vi "6704_set_static_voltages.vi"(6 "error in":errorcluster, 8 "6704 Static Voltage Settings":T1={"Device Name"="6704_Static", "Values"=[5.0, 0.0, 0.0, 0.0, 0.0, 0.0, 0.0, 0.0, 0.0, 0.0, 0.0, 0.0, 0.0, 0.0, 0.0, 0.0], "Nickname"=["", "", "", "", "", "", "", "", "", "", "", "", "", "", "", ""], "Conversion"=[enum."Volts", enum."Volts", enum."Volts", enum."Volts", enum."Volts", enum."Volts", enum."Volts", enum."Volts", enum."Volts", enum."Volts", enum."Volts", enum."Volts", enum."Volts", enum."Volts", enum."Volts", enum."Volts"]}) -> (0 "error out":errorcluster, 2 "Voltages Out":dbl[](array[numeric]))   [LabVIEW 2015]
uses:
  Controls/6704/6704_static_voltages_control.ctl
  Controls/6704/static_voltage_conversions.ctl
  Controls/6704/6704_state_machine_enum.ctl
  <vilib>/DAQmx/write.llb/DAQmx Write (Analog 1D DBL NChan 1Samp).vi
  <vilib>/DAQmx/create/channels.llb/DAQmx Create Channel (AO-Voltage-Basic).vi
  <vilib>/DAQmx/miscellaneous.llb/DAQmx Fill In Error Info.vi
  <resource>/objmgr/daqmx.rc
panel:
  out "AO.Voltage.Rngs":dbl[](array[numeric])
  out "Active Device":tag
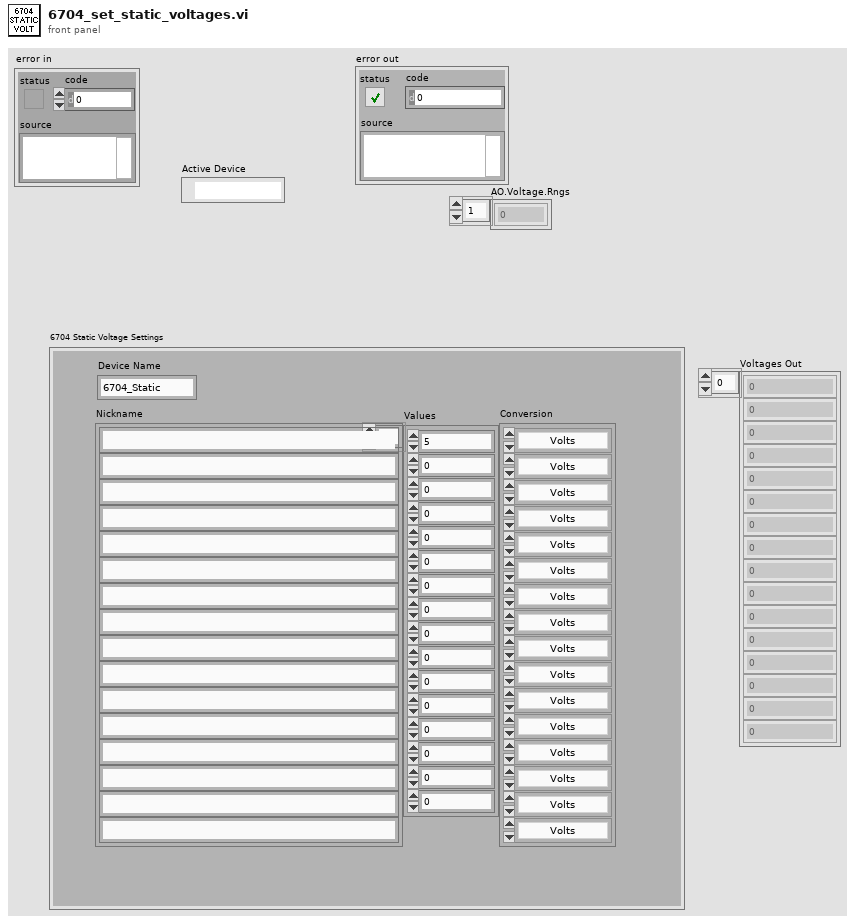
[diagram p1: front panel]
types:
  T1 = typedef "6704_static_voltages_control.ctl" = cluster{"Device Name":string, "Values":dbl[], "Nickname":string[], "Conversion":T2[]}
  T2 = typedef "static_voltage_conversions.ctl" = enum16{"Volts", "ODT Power Lock (W)", "Sat Abs Detuning (MHz)", "Blue Mot Power Lock (mW)"}
  T3 = typedef "6704_state_machine_enum.ctl" = enum16{"Initialize", "Convert to Voltage", "Set Voltages", "Debug"}
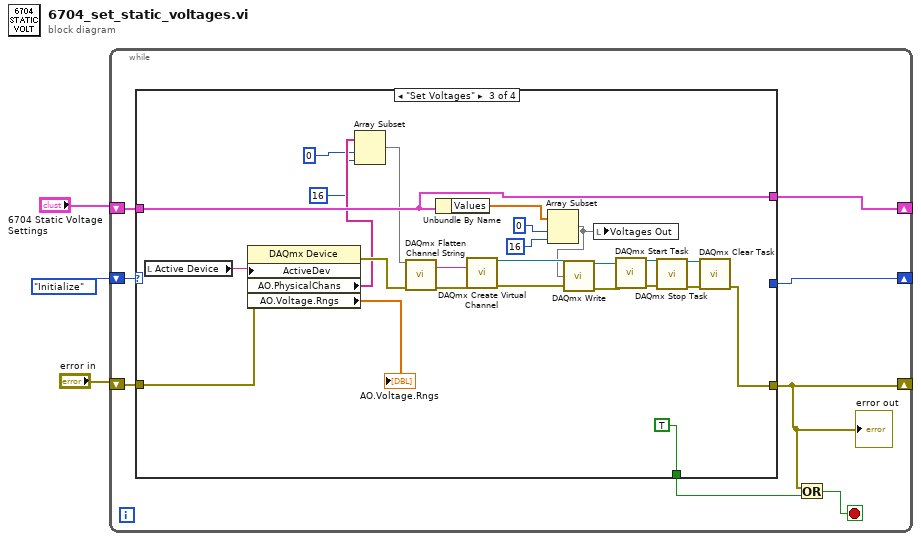
[diagram p0: block diagram]
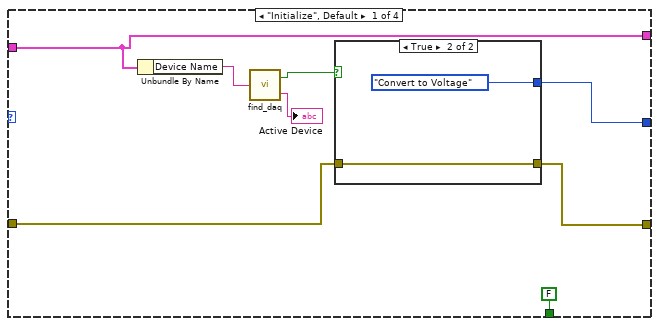
[diagram p2: hidden frame]
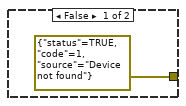
[diagram p3: hidden frame]
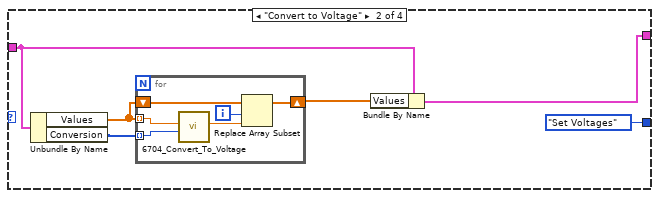
[diagram p4: hidden frame]
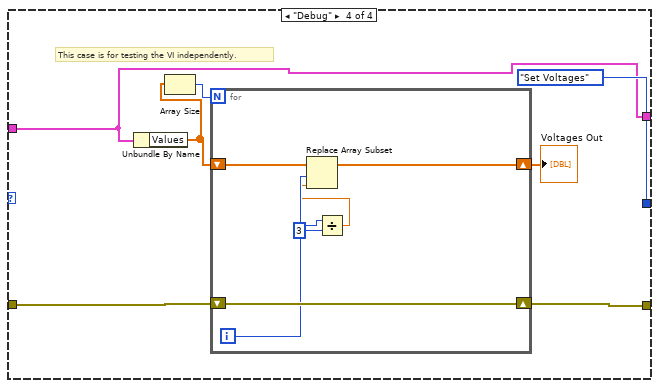
[diagram p5: hidden frame]
diagram:
  n1 = while {
    shift-right: [w4] -> _
    shift-left: "error in" -> [w9]
    shift-right: [w8] -> _
    shift-left: 6704_state_machine_enum."Initialize" -> [w11]
    shift-right: [w6] -> _
    shift-left: "6704 Static Voltage Settings" -> [w10]
    stop <- w7 stop-if-true
    n2 = case shown="\"Set Voltages\"" w11 {
      tunnel: w10 -> [w13 w25 w50 w60]
      tunnel: w9 -> [w14 _ w59 w65]
      tunnel: [w16 6704_state_machine_enum."Set Voltages" _ 6704_state_machine_enum."Set Voltages"] -> w8
      tunnel: [w15 _ w53 w66] -> w4
      tunnel: [w13 w24 w50 w60] -> w6
      tunnel: [FALSE ("y") _ TRUE ("y") _] -> w5
      frame "Initialize", Default {
        n3 = Unbundle By Name(w13) -> ("Device Name"=w19:string)
        n4 = call "find_daq.vi"("Device Name"=w19) -> ("Device Present"=w18:bool, "DAQmx Device Name"=→"Active Device":tag)
        n5 = case shown="True" w18 {
          tunnel: [_ 6704_state_machine_enum."Convert to Voltage"] -> w16
          tunnel: [errorcluster {"status"=TRUE, "code"=1, "source"="Device not found"} ("error in") w21] -> w15
          tunnel: w14 -> [_ w21]
          frame False {
          }
          frame True {
          }
        }
      }
      frame "Convert to Voltage" {
        n6 = Unbundle By Name(w25) -> ("Values"=w27:dbl[], "Conversion"=w28:T2[])
        n7 = for {
          tunnel: w27 -> [w34] mode=indexing
          tunnel: w28 -> [w33] mode=indexing
          shift-right: [w30] -> w26
          shift-left: w27 -> [w29]
          i -> [w31]
          n8 = call "6704_Convert_To_Voltage.vi"("Conversion"=w33, "Value"=w34) -> ("Voltage"=w32:dbl)  [unwired: 9 in]
          n9 = Replace Array Subset(array=w29, new element=w32, index=w31) -> (w30:dbl[])
        }
        n10 = Bundle By Name(cluster=w25, "Values"=w26) -> (w24:T1)
      }
      frame "Set Voltages" {
        n11 = local read "Active Device"() -> (w58:tag)
        n12 = property class="DAQmx Device"(error in=w59, "ActiveDev"=w58) -> (error out=w48:errorcluster, "AO.PhysicalChans"=w44:tag[], "AO.Voltage.Rngs"=→"AO.Voltage.Rngs":dbl[])  [unwired: 1 in, 1 out]
        n13 = Array Subset(array=w44, index=0, length=16) -> (w41:tag[])
        n14 = call <vilib>:"DAQmx Flatten Channel String.vi"("names in"=w41, "error in"=w48) -> ("names out"=w49:string, "error out"=w47:errorcluster)  [unwired: 12 in]
        n15 = Unbundle By Name(w50) -> ("Values"=w37:dbl[])
        n16 = call-poly <vilib>:"DAQmx Create Virtual Channel.vi"("physical channels"=w49, "error in"=w47) -> ("task out"=w40:refnum<k21>, "error out"=w57:errorcluster)  [unwired: 12 in]
        n17 = Array Subset(array=w37, index=0, length=16) -> (w36:dbl[])
        n18 = call-poly <vilib>:"DAQmx Write.vi"("task/channels in"=w40, "data"=w36, "error in"=w57) -> ("task out"=w56:refnum<k21>, "error out"=w55:errorcluster)  [unwired: 10 in, 1 out]
        n19 = local write "Voltages Out"(w36) -> ()
        n20 = call <vilib>:"DAQmx Start Task.vi"("task/channels in"=w56, "error in"=w55) -> ("task out"=w38:refnum<k21>, "error out"=w39:errorcluster)  [unwired: 12 in]
        n21 = call <vilib>:"DAQmx Stop Task.vi"("task/channels in"=w38, "error in"=w39) -> ("task out"=w52:refnum<k21>, "error out"=w54:errorcluster)  [unwired: 12 in]
        n22 = call <vilib>:"DAQmx Clear Task.vi"("task in"=w52, "error in"=w54) -> ("error out"=w53:errorcluster)  [unwired: 13 in]
      }
      frame "Debug" {
        # "This case is for testing the VI independently."
        n23 = Unbundle By Name(w60) -> ("Values"=w61:dbl[])
        n24 = Array Size(array=w61) -> (size(s)=w62:i32)
        n25 = for {
          N: w62 -> [_]
          shift-right: [w72] -> w66
          shift-left: w65 -> [w72]
          shift-right: [w70] -> w64
          shift-left: w61 -> [w71]
          i -> [w69]
          n26 = Divide(x=w69, y=3) -> (x/y=w67:dbl)
          n27 = Replace Array Subset(array=w71, new element=w67, index=w69) -> (w70:dbl[])
        }
        "Voltages Out" <- w64
      }
    }
    "error out" <- w4
    n28 = Or(x=w4, y=w5) -> (x .or. y?=w7:bool)
  }
